vi "CloseAllPorts.vi"   [LabVIEW 2012]
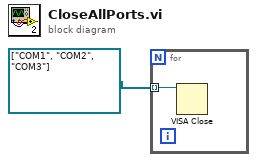
[diagram p0: block diagram]
diagram:
  n1 = for {
    tunnel: refnum<visa-resource-name>[] ["COM1", "COM2", "COM3"] -> [w2] mode=indexing
    n2 = VISA Close(VISA resource name=w2) -> ()  [unwired: 1 in, 1 out]
  }
